vi "Pre Launch Init.vi"(11 "Table View in":refnum<class "Table View.lvclass">) -> (0 "error out":errorcluster, 3 "Table View out":refnum<class "Table View.lvclass">)   [LabVIEW 2020, in "[V]Table View.lvlib" / "Table View.lvclass"]
doc: "(<B>Filename</B>: Actor Framework.lvlib:Actor.lvclass:Pre Launch Init.vi)\n\nDefines behavior that occurs after the Launch Nested Actor method is invoked but before the actor's Actor Core method begins running.\n\nBy default, this method does nothing. A descendant class may override it to define behavior."
uses:
  Table View.lvclass
  MVVM Framework/MVVM Abstruct View/MVVM Abstruct View/MVVM Abstruct View.lvclass
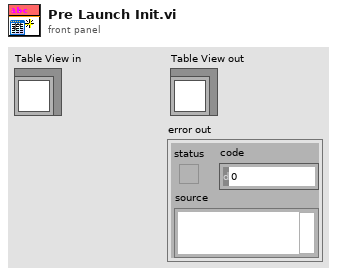
[diagram p1: front panel]
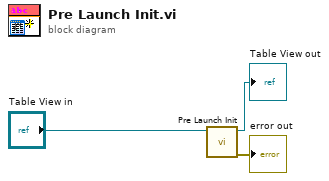
[diagram p0: block diagram]
diagram:
  n1 = call-parent "Pre Launch Init.vi"("Abstruct View in"="Table View in") -> ("error out"=→"error out":errorcluster, "Abstruct View out"=→"Table View out":refnum<class "Table View.lvclass">)  [unwired: 9 in]
